vi "numerical-integration-test.vi"() -> (3 "All passed":bool)   [LabVIEW 2019]
uses:
  <vilib>/Analysis/Matrix/Datatypes/RealMatrix.ctl
  <vilib>/Rock Robotics/WPI/ThirdParty/JAS_Junk/TrajLib/MatBuilder_Create.vi
  <vilib>/Rock Robotics/WPI/ThirdParty/JAS_Junk/TrajLib/Trajectory_Library.lvlib
  <vilib>/Analysis/Matrix/NI_Matrix.lvlib
panel:
  out "Passed 1":bool
  out "Error 1":bool
  out "Test 1":T1
  out "Passed  0":bool
  out "Error 0":bool
  out "Test 0":T1
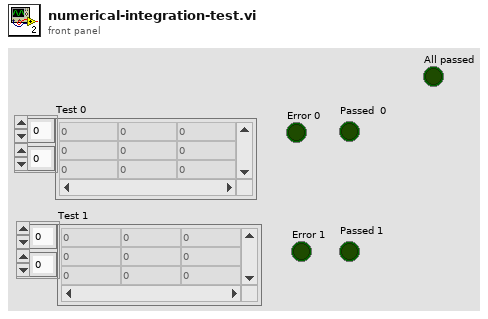
[diagram p1: front panel]
types:
  T1 = typedef "NI_Matrix.lvlib/RealMatrix.ctl" = dbl[][]
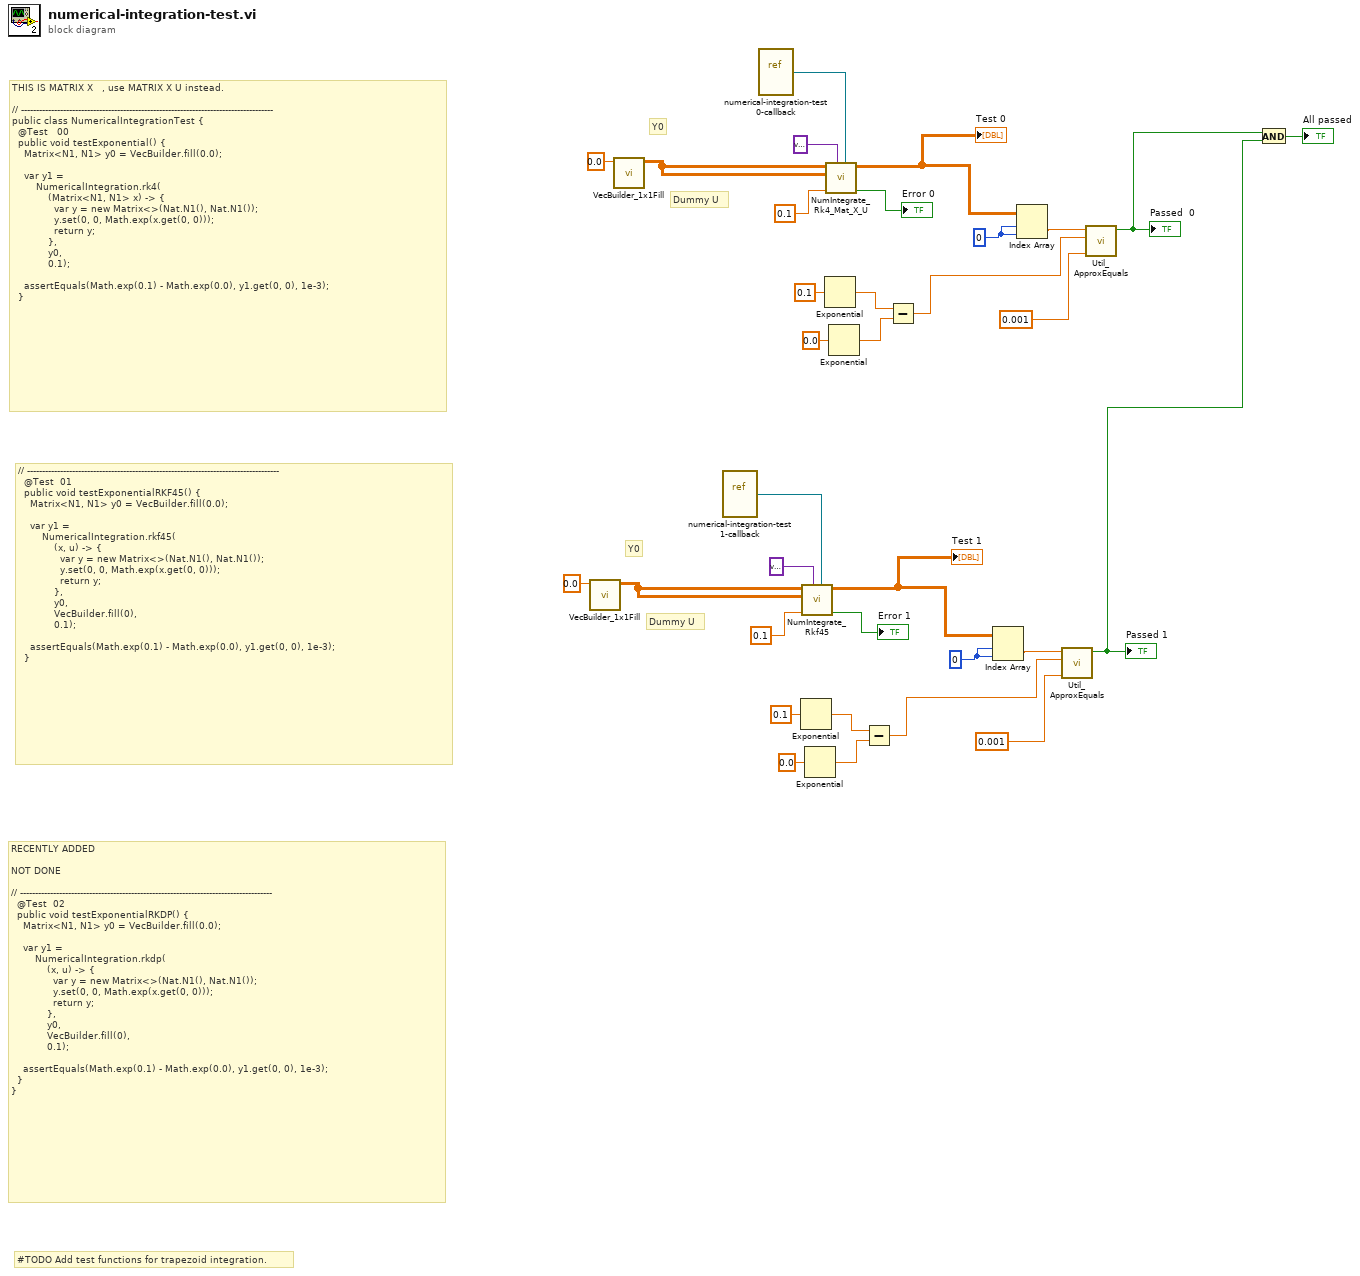
[diagram p0: block diagram]
diagram:
  w13 = 0 ("index (row)")
  w27 = 0 ("index (row)")
  # "#TODO Add test functions for trapezoid integration."
  # "Dummy U"
  # "Y0"
  # "Dummy U"
  # "Y0"
  # "// ------------------------------------------------------------------------------------\n  @Test  01\n  public void testExponentialRKF45() {\n    Matrix<N1, N1> y0 = VecBuilder.fill(0.0);\n\n    var y1 =\n        NumericalIntegration.rkf45(\n            (x, u) -> {\n              var y = new Matrix<>(Nat.N1(), Nat.N1());\n              y.set(0, 0, Math.exp(x.get(0, 0)));\n              return y;\n            },\n            y0,\n            VecBuilder.fill(0),\n            0.1);\n\n    assertEquals(Math.exp(0.1) - Math.exp(0.0), y1.get(0, 0), 1e-3);\n  }"
  # "THIS IS MATRIX X   , use MATRIX X U instead.\n\n// ------------------------------------------------------------------------------------\npublic class NumericalIntegrationTest {\n  @Test   00\n  public void testExponential() {\n    Matrix<N1, N1> y0 = VecBuilder.fill(0.0);\n\n    var y1 =\n        NumericalIntegration.rk4(\n            (Matrix<N1, N1> x) -> {\n              var y = new Matrix<>(Nat.N1(), Nat.N1());\n              y.set(0, 0, Math.exp(x.get(0, 0)));\n              return y;\n            },\n            y0,\n            0.1);\n\n    assertEquals(Math.exp(0.1) - Math.exp(0.0), y1.get(0, 0), 1e-3);\n  }"
  # "RECENTLY ADDED\n\nNOT DONE\n\n// ------------------------------------------------------------------------------------\n  @Test  02\n  public void testExponentialRKDP() {\n    Matrix<N1, N1> y0 = VecBuilder.fill(0.0);\n\n    var y1 =\n        NumericalIntegration.rkdp(\n            (x, u) -> {\n              var y = new Matrix<>(Nat.N1(), Nat.N1());\n              y.set(0, 0, Math.exp(x.get(0, 0)));\n              return y;\n            },\n            y0,\n            VecBuilder.fill(0),\n            0.1);\n\n    assertEquals(Math.exp(0.1) - Math.exp(0.0), y1.get(0, 0), 1e-3);\n  }\n}"
  n1 = call <vilib>:"VecBuilder_1x1Fill.vi"("R0_C0"=0.0) -> ("output matrix"=w16:T1)  [unwired: 10 in]
  n2 = call <vilib>:"VecBuilder_1x1Fill.vi"("R0_C0"=0.0) -> ("output matrix"=w31:T1)  [unwired: 10 in]
  n3 = vi-ref "numerical-integration-test1-callback.vi"() -> (w1:refnum<vi>)
  n4 = vi-ref "numerical-integration-test0-callback.vi"() -> (w28:refnum<vi>)
  n5 = Exponential(1:0.1 ("x")) -> (0:w6:dbl)
  n6 = call <vilib>:"NumIntegrate_Rkf45.vi"("NumInt_RKF45_Func_Type"=w1, "PassedData"=variant, "dT_Seconds"=0.1, "U"=w16, "X"=w16) -> ("Error"=→"Error 1":bool, "Return X"=w12:T1)  [unwired: 4 in, 1 out]
  "Test 1" <- w12
  n7 = Exponential(1:0.0 ("x")) -> (0:w5:dbl)
  n8 = Exponential(1:0.1 ("x")) -> (0:w20:dbl)
  n9 = call <vilib>:"NumIntegrate_Rk4_Mat_X_U.vi"("NumInt_RK4_Func_Type"=w28, "PassedData"=variant, "dT_Seconds"=0.1, "U"=w31, "X"=w31) -> ("Error"=→"Error 0":bool, "OUTPUT"=w26:T1)  [unwired: 5 in]
  "Test 0" <- w26
  n10 = Exponential(1:0.0 ("x")) -> (0:w19:dbl)
  n11 = Subtract(x=w6, y=w5) -> (x-y=w7:dbl)
  n12 = Subtract(x=w20, y=w19) -> (x-y=w21:dbl)
  n13 = Index Array(array=w12, index (row)=w13, index (col)=w13) -> (element=w10:dbl)
  n14 = Index Array(array=w26, index (row)=w27, index (col)=w27) -> (element=w24:dbl)
  n15 = call "Util_ApproxEquals.vi"("Tolerance"=0.001, "Value 2"=w7, "Value 1"=w10) -> ("ApproxEquals"=w3:bool)  [unwired: 8 in]
  "Passed 1" <- w3
  n16 = call "Util_ApproxEquals.vi"("Tolerance"=0.001, "Value 2"=w21, "Value 1"=w24) -> ("ApproxEquals"=w4:bool)  [unwired: 8 in]
  "Passed  0" <- w4
  n17 = And(x=w4, y=w3) -> (x .and. y?=→"All passed":bool)
